vi "sub clear_leds.vi"() -> (0 "String":string)   [LabVIEW 2016]
uses:
  ledmatrix_default.ctl
panel:
  in  "Array 2":T1
  out "output array":u8[](array[numeric])
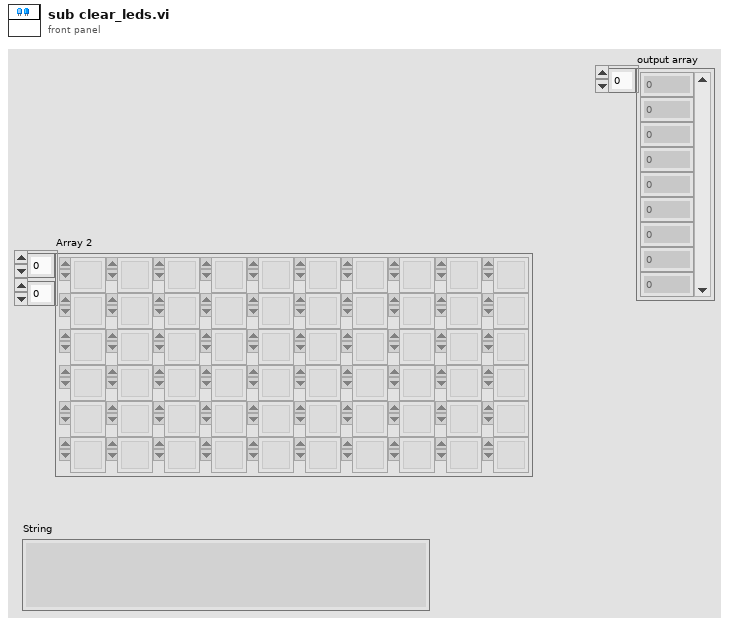
[diagram p1: front panel]
types:
  T1 = typedef "ledmatrix_default.ctl" = u8[][]
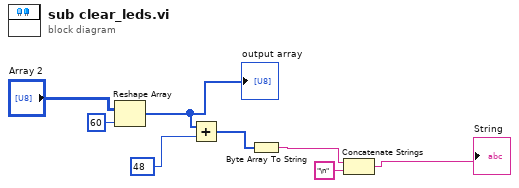
[diagram p0: block diagram]
diagram:
  n1 = Reshape Array("Array 2", 60 ("dimension size")) -> (w4:u8[])
  "output array" <- w4
  n2 = Add(x=w4, y=u8 48 ("dimension size")) -> (x+y=w2:u8[])
  n3 = Byte Array To String(unsigned byte array=w2) -> (string=w7:string)
  n4 = Concatenate Strings(w7, "\n" ("string")) -> (→"String":string)
